vi "Test_Cache.vi"() -> ()   [LabVIEW 2020]
uses:
  ClassLoader.lvlib
panel:
  out "error out":errorcluster
  in  "error in":errorcluster
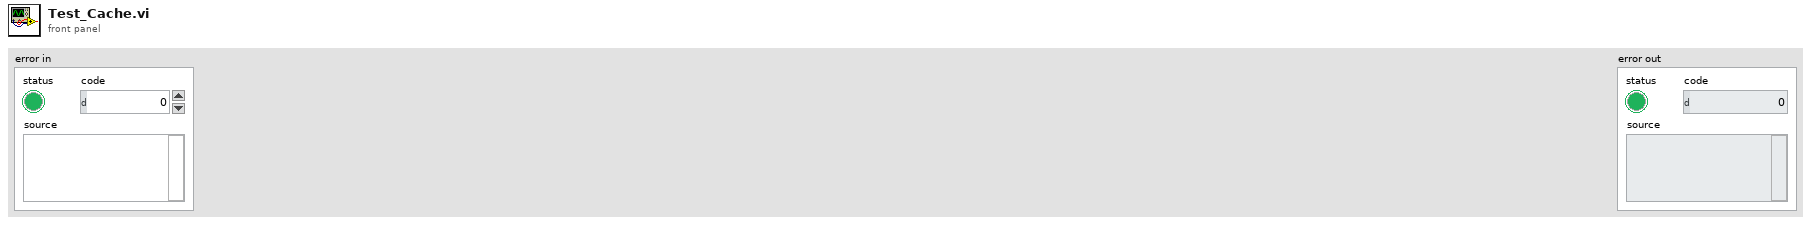
[diagram p1: front panel]
types:
  T1 = typedef "ClassLoader.lvlib/Ctl_PPL Details Cluster.ctl" = cluster{"Name":string, "Path":path, "Version":string}
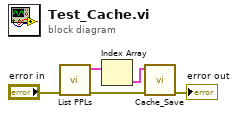
[diagram p0: block diagram]
diagram:
  n1 = call "List PPLs.vi"("error in"="error in") -> ("error out"=w1:errorcluster, "PPL Details"=w5:T1[])  [unwired: 8 in, 1 out]
  n2 = Index Array(array=w5) -> (element=w3:T1)  [unwired: 1 in]
  n3 = call "Cache_Save.vi"("error in"=w1, "PPL Details"=w3) -> ("error out"=→"error out":errorcluster)  [unwired: 7 in, 2 out]
